vi "运维调试.vi"() -> ()   [LabVIEW 2016]
uses:
  <vilib>/Utility/miscctls.llb/LVPointTypeDef.ctl
  PLC/PLC.lvlib
  API/CodCr/CodCr.lvlib
  <vilib>/Utility/config.llb/NI_LVConfig.lvlib
panel:
  out "数值":i32
  in  "运维调试菜单":T1(xcontrol)
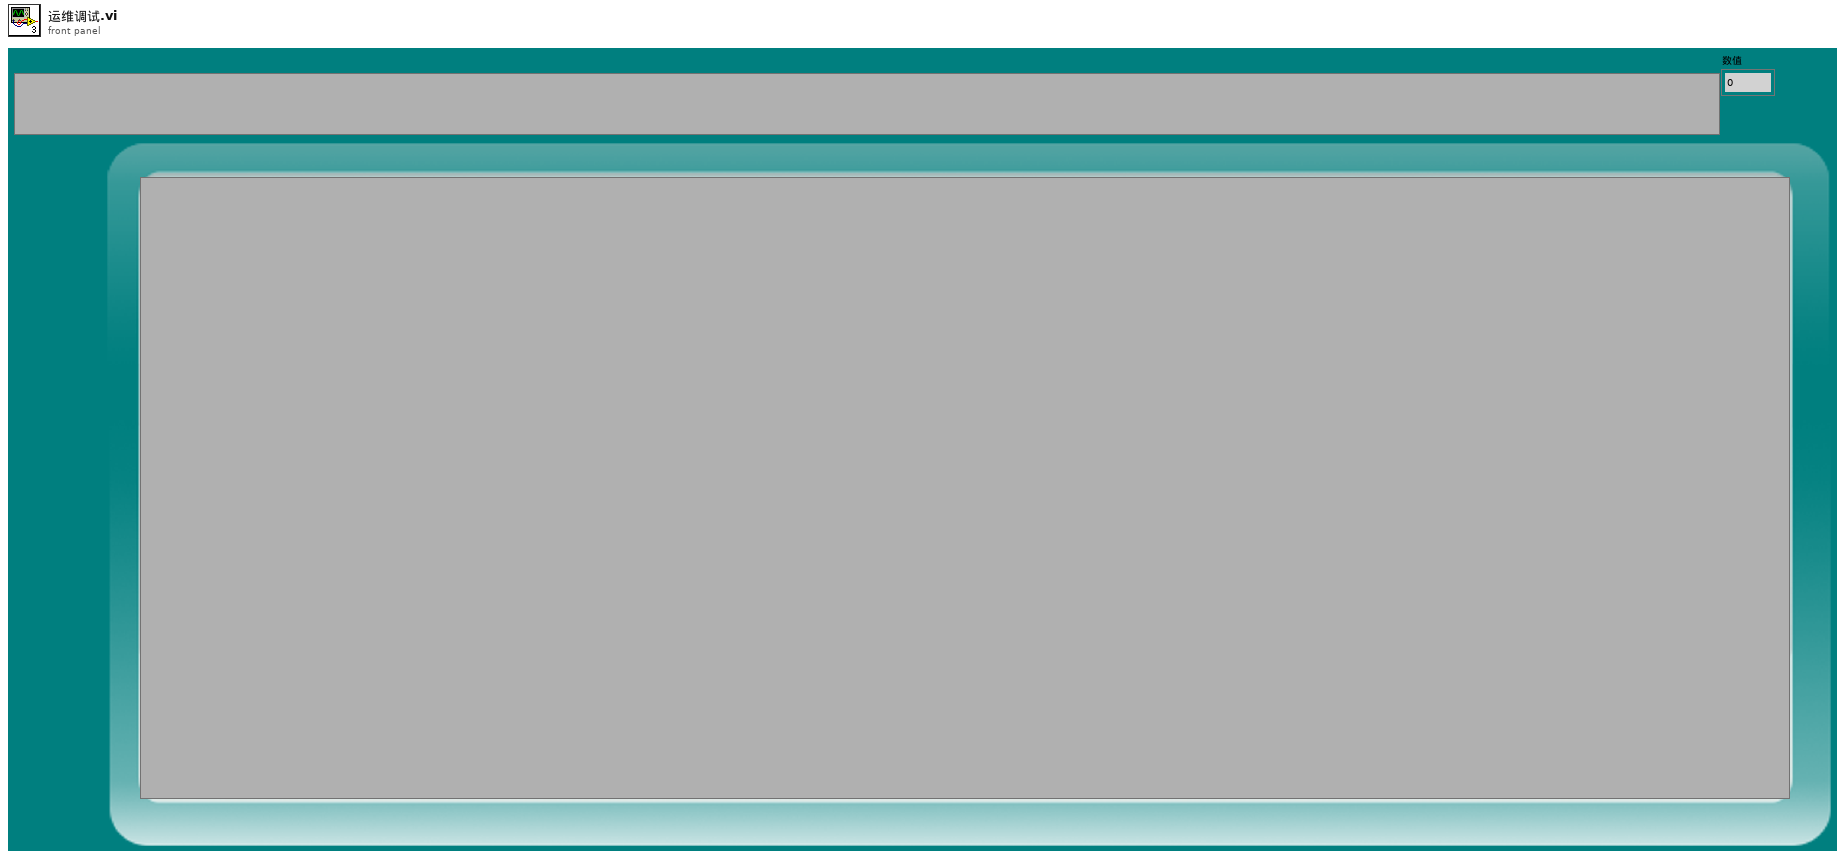
[diagram p1: front panel]
types:
  T1 = enum16{"电源管理", "采配水", "氨氮", "总磷总氮", "多参数", "CODMn", "CODcr", "流量计", "质控单元", "其他"}
  T2 = typedef "NI_LVConfig.lvlib/Config Data RefNum.ctl" = refnum<k1>
  T3 = typedef "LVPointTypeDef.ctl" = cluster{"Horizontal":i16, "Vertical":i16}
  T4 = enum16{"Enabled", "Disabled", "Disabled and Grayed Out"}
  T5 = enum32{"Bad", "Idle", "Run top level", "Running"}
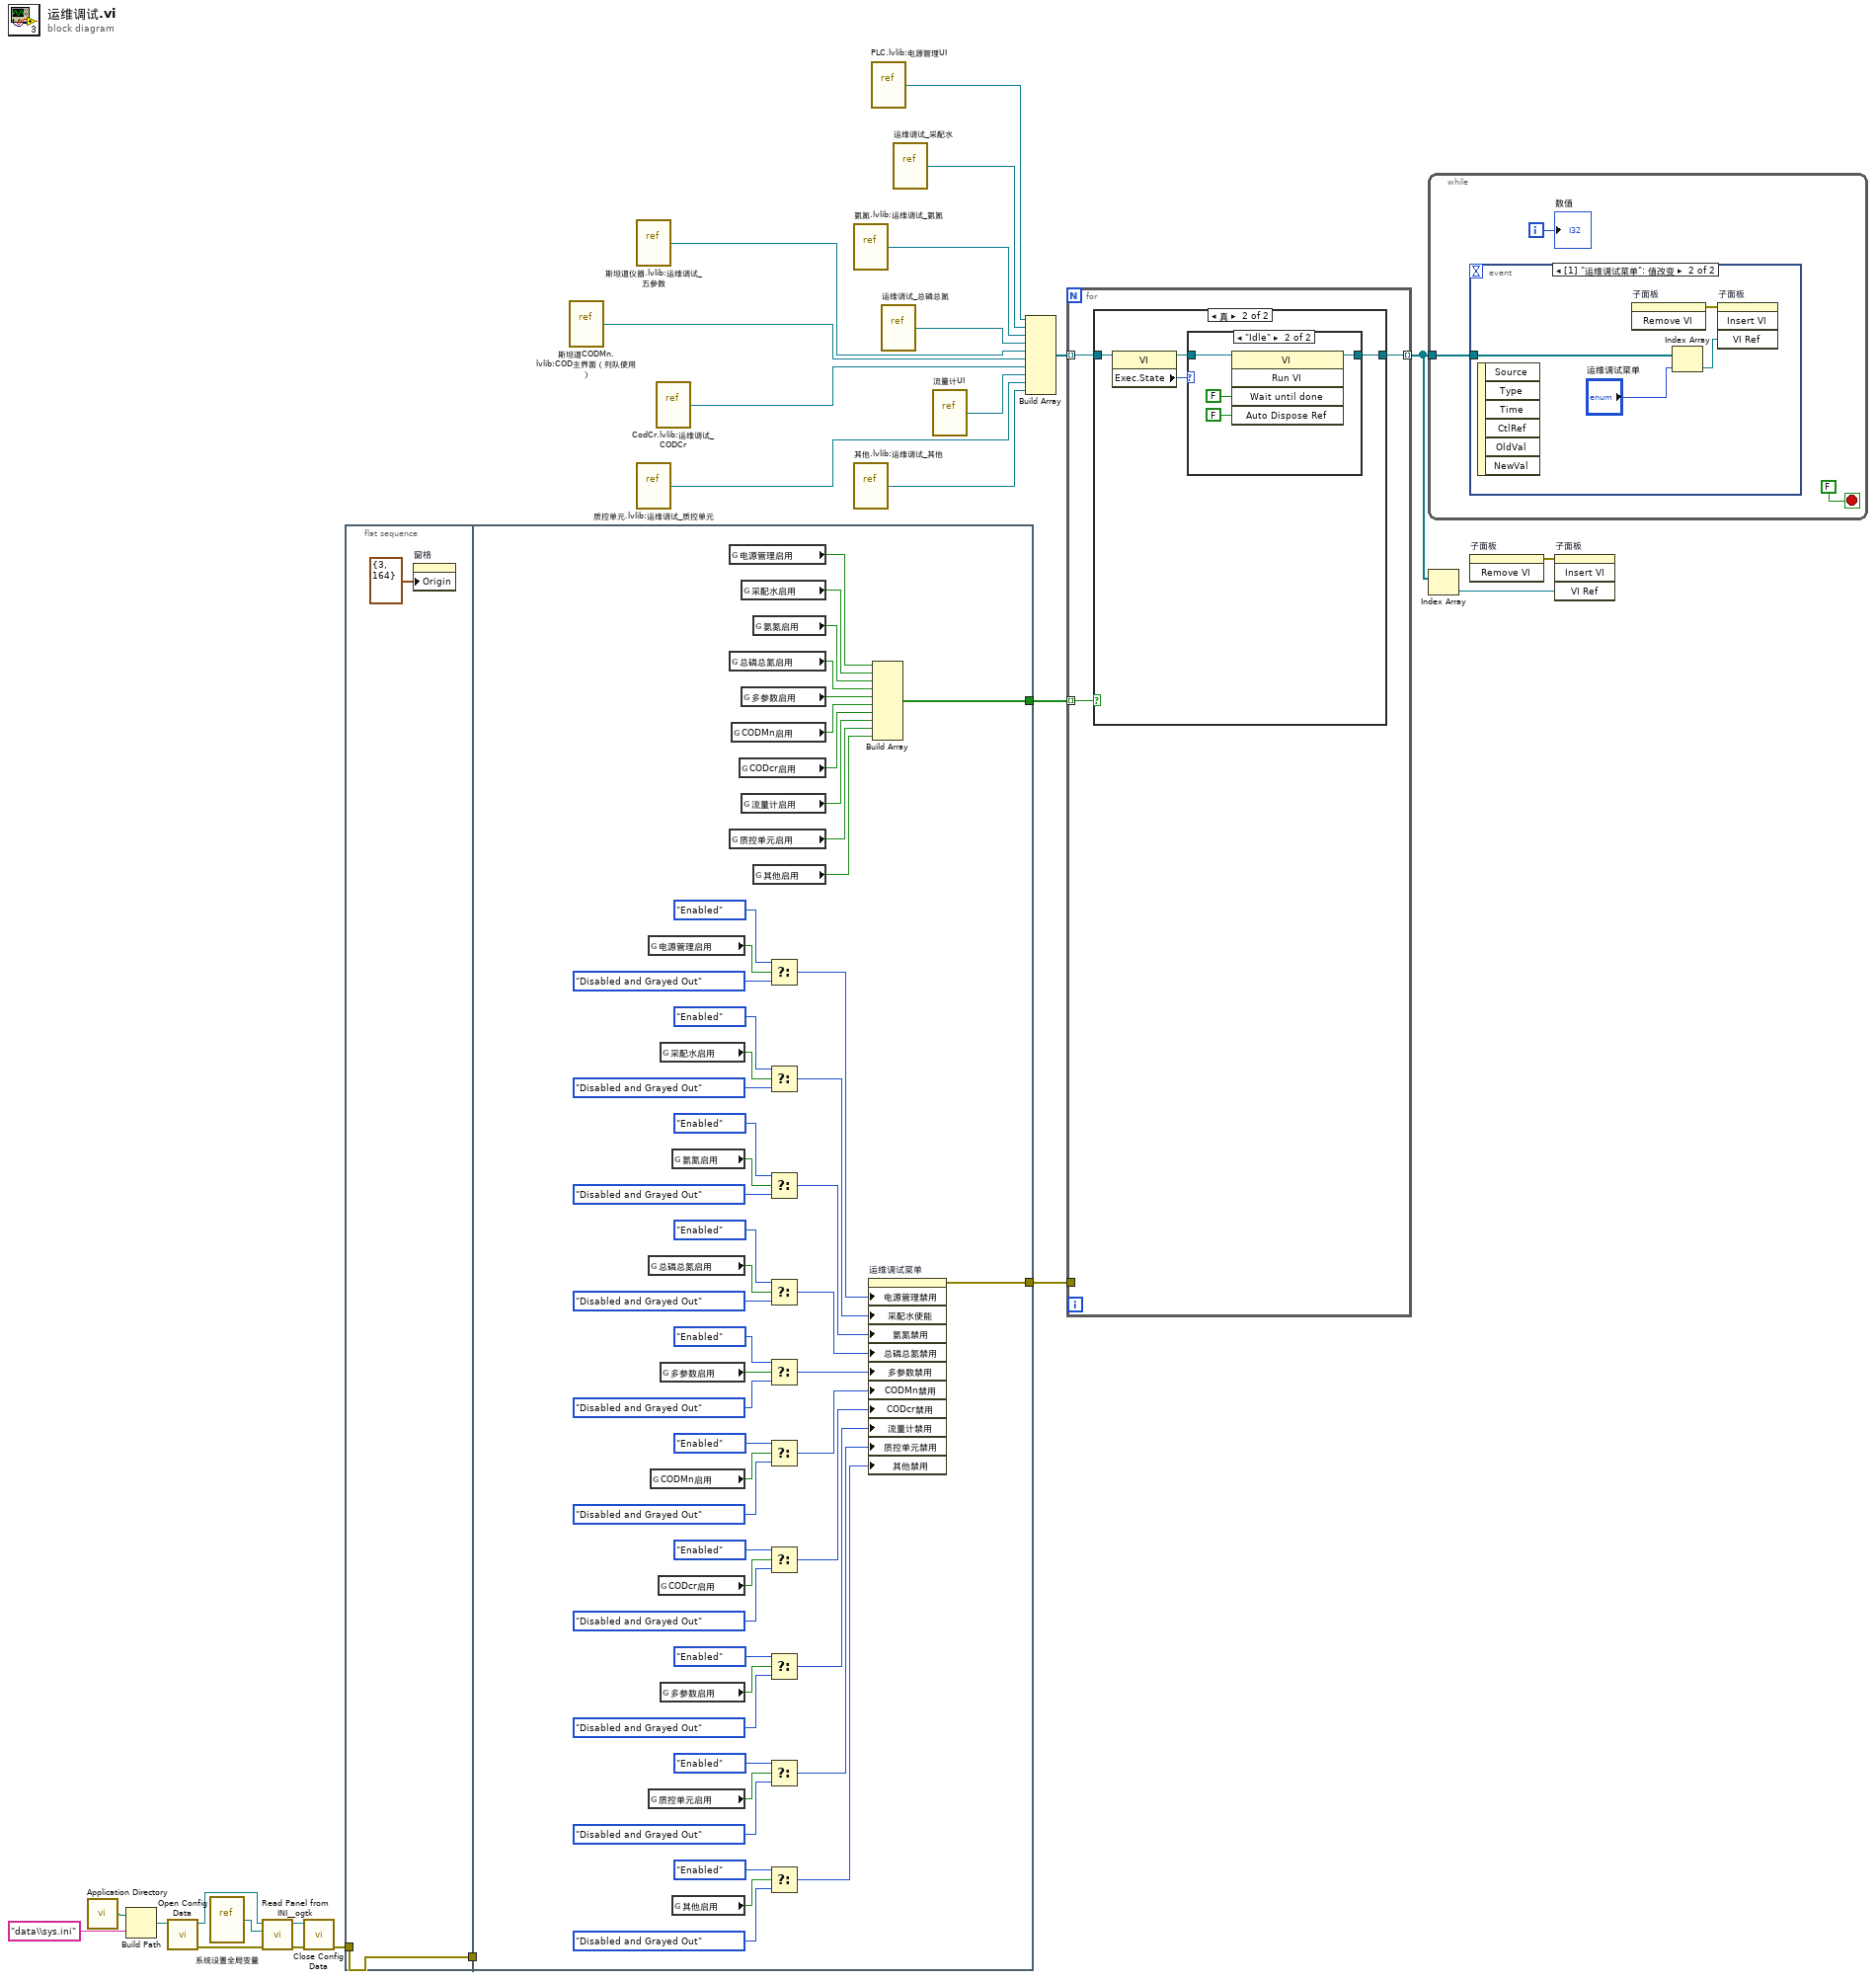
[diagram p0: block diagram]
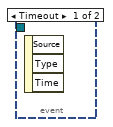
[diagram p4: hidden frame]
diagram:
  n1 = call <vilib>:"Application Directory.vi"() -> ("Application Directory"=w4:path)
  n2 = Build Path(base path=w4, name or relative path="data\\sys.ini" ("名称或相对路径")) -> (appended path=w2:path)
  n3 = call <vilib>:"Open Config Data.vi"("configuration file path"=w2) -> ("error out"=w11:errorcluster, "refnum"=w10:T2)  [unwired: 8 in, 1 out]
  n4 = vi-ref "系统设置全局变量.vi"() -> (w9:refnum<vi>)
  n5 = call <userlib>:"Read Panel from INI__ogtk.vi"("error in (no error)"=w11, "VI ref"=w9, "refnum"=w10) -> ("error out"=w8:errorcluster, "refnum out"=w7:T2)  [unwired: 7 in]
  n6 = call <vilib>:"Close Config Data.vi"("error in (no error)"=w8, "refnum"=w7) -> ("error out"=w6:errorcluster)  [unwired: 8 in, 1 out]
  n7 = flat-sequence {
    tunnel: w6 -> [w28]
    tunnel: [w28] -> w5
    tunnel: [w60] -> w12
    tunnel: w5 -> [_]
    tunnel: [w49] -> w1
    frame #0 {
      n8 = property on="窗格" class="Pane"("Origin"=T3 {"Horizontal"=3, "Vertical"=164} ("原点")) -> ()  [unwired: 2 in, 2 out]
    }
    frame #1 {
      n9 = global read "系统设置全局变量.vi" "电源管理启用"() -> (w80:bool)
      n10 = global read "系统设置全局变量.vi" "总磷总氮启用"() -> (w74:bool)
      n11 = global read "系统设置全局变量.vi" "质控单元启用"() -> (w67:bool)
      n12 = global read "系统设置全局变量.vi" "CODMn启用"() -> (w70:bool)
      n13 = global read "系统设置全局变量.vi" "CODcr启用"() -> (w69:bool)
      n14 = global read "系统设置全局变量.vi" "采配水启用"() -> (w77:bool)
      n15 = global read "系统设置全局变量.vi" "多参数启用"() -> (w72:bool)
      n16 = global read "系统设置全局变量.vi" "多参数启用"() -> (w68:bool)
      n17 = global read "系统设置全局变量.vi" "氨氮启用"() -> (w76:bool)
      n18 = global read "系统设置全局变量.vi" "其他启用"() -> (w66:bool)
      n19 = global read "系统设置全局变量.vi" "电源管理启用"() -> (w50:bool)
      n20 = global read "系统设置全局变量.vi" "总磷总氮启用"() -> (w53:bool)
      n21 = global read "系统设置全局变量.vi" "质控单元启用"() -> (w58:bool)
      n22 = global read "系统设置全局变量.vi" "CODMn启用"() -> (w55:bool)
      n23 = global read "系统设置全局变量.vi" "CODcr启用"() -> (w56:bool)
      n24 = global read "系统设置全局变量.vi" "采配水启用"() -> (w51:bool)
      n25 = global read "系统设置全局变量.vi" "多参数启用"() -> (w54:bool)
      n26 = global read "系统设置全局变量.vi" "流量计启用"() -> (w57:bool)
      n27 = global read "系统设置全局变量.vi" "氨氮启用"() -> (w52:bool)
      n28 = global read "系统设置全局变量.vi" "其他启用"() -> (w59:bool)
      n29 = Select(t=T4."Enabled" ("电源管理禁用"), s=w80, f=T4."Disabled and Grayed Out" ("电源管理禁用")) -> (s? t:f=w79:T4)
      n30 = Select(t=T4."Enabled" ("电源管理禁用"), s=w77, f=T4."Disabled and Grayed Out" ("电源管理禁用")) -> (s? t:f=w78:T4)
      n31 = Select(t=T4."Enabled" ("电源管理禁用"), s=w76, f=T4."Disabled and Grayed Out" ("电源管理禁用")) -> (s? t:f=w75:T4)
      n32 = Select(t=T4."Enabled" ("电源管理禁用"), s=w74, f=T4."Disabled and Grayed Out" ("电源管理禁用")) -> (s? t:f=w73:T4)
      n33 = Select(t=T4."Enabled" ("电源管理禁用"), s=w72, f=T4."Disabled and Grayed Out" ("电源管理禁用")) -> (s? t:f=w71:T4)
      n34 = Select(t=T4."Enabled" ("电源管理禁用"), s=w70, f=T4."Disabled and Grayed Out" ("电源管理禁用")) -> (s? t:f=w65:T4)
      n35 = Select(t=T4."Enabled" ("电源管理禁用"), s=w69, f=T4."Disabled and Grayed Out" ("电源管理禁用")) -> (s? t:f=w64:T4)
      n36 = Select(t=T4."Enabled" ("电源管理禁用"), s=w68, f=T4."Disabled and Grayed Out" ("电源管理禁用")) -> (s? t:f=w63:T4)
      n37 = Select(t=T4."Enabled" ("电源管理禁用"), s=w67, f=T4."Disabled and Grayed Out" ("电源管理禁用")) -> (s? t:f=w62:T4)
      n38 = Select(t=T4."Enabled" ("电源管理禁用"), s=w66, f=T4."Disabled and Grayed Out" ("电源管理禁用")) -> (s? t:f=w61:T4)
      n39 = property on="运维调试菜单" class="运维调试菜单 (严格)"("电源管理禁用"=w79, "采配水使能"=w78, "氨氮禁用"=w75, "总磷总氮禁用"=w73, "多参数禁用"=w71, "CODMn禁用"=w65, "CODcr禁用"=w64, "流量计禁用"=w63, "质控单元禁用"=w62, "其他禁用"=w61) -> (error out=w60:errorcluster)  [unwired: 2 in, 1 out]
      n40 = Build Array(w50, w51, w52, w53, w54, w55, w56, w57, w58, w59) -> (w49:bool[])
    }
  }
  n41 = vi-ref "斯坦道CODMn.lvlib:COD主界面（列队使用）.vi"() -> (w18:refnum<vi>)
  n42 = vi-ref "斯坦道仪器.lvlib:运维调试_五参数.vi"() -> (w19:refnum<vi>)
  n43 = vi-ref "质控单元.lvlib:运维调试_质控单元.vi"() -> (w16:refnum<vi>)
  n44 = vi-ref "CodCr.lvlib:运维调试_CODCr.vi"() -> (w17:refnum<vi>)
  n45 = vi-ref "氨氮.lvlib:运维调试_氨氮.vi"() -> (w21:refnum<vi>)
  n46 = vi-ref "其他.lvlib:运维调试_其他.vi"() -> (w15:refnum<vi>)
  n47 = vi-ref "PLC.lvlib:电源管理UI.vi"() -> (w14:refnum<vi>)
  n48 = vi-ref "运维调试_总磷总氮.vi"() -> (w20:refnum<vi>)
  n49 = vi-ref "运维调试_采配水.vi"() -> (w22:refnum<vi>)
  n50 = vi-ref "流量计UI.vi"() -> (w13:refnum<vi>)
  n51 = Build Array(w14, w22, w21, w20, w19, w18, w17, w13, w16, w15) -> (w23:refnum<vi>[])
  n52 = for {
    tunnel: w23 -> [w83] mode=indexing
    tunnel: [w82] -> w25 mode=indexing
    tunnel: w1 -> [w81] mode=indexing
    tunnel: w12 -> [_]
    n53 = case shown="真" w81 {
      tunnel: w83 -> [w84 w88]
      tunnel: [w84 w85] -> w82
      frame False {
      }
      frame True {
        n54 = property class="VI"(reference=w88) -> (reference out=w86:refnum<vi>, "Exec.State"=w87:T5)  [unwired: 1 in, 1 out]
        n55 = case shown="\"Idle\"" w87 {
          tunnel: w86 -> [w89 w91]
          tunnel: [w89 w90] -> w85
          frame "Bad", Default {
          }
          frame "Idle" {
            n56 = invoke class="VI" method="Run VI"(reference=w91, "Wait until done"=FALSE ("结束前等待"), "Auto Dispose Ref"=FALSE ("自动销毁引用")) -> (reference out=w90:refnum<vi>)  [unwired: 2 in, 4 out]
          }
        }
      }
    }
  }
  n57 = while {
    tunnel: w25 -> [w95]
    i -> [w94]
    stop <- FALSE stop-if-true
    n58 = event shown="[1] \"运维调试菜单\": 值改变" {
      selector: _ -> [_ _]
      dyn-events: _ -> [_ _]
      timeout: _ -> [_ _]
      tunnel: w95 -> [_ w99]
      event Timeout {
        n59 = event-data() -> ()  [unwired: 1 in, 3 out]
      }
      event "运维调试菜单": Value Change {
        n60 = event-data() -> ()  [unwired: 1 in, 6 out]
        n61 = invoke on="子面板" class="SubPnl" method="Remove VI"() -> (error out=w100:errorcluster)  [unwired: 3 in, 2 out]
        n62 = Index Array(array=w99, index="运维调试菜单") -> (element=w98:refnum<vi>)
        n63 = invoke on="子面板" class="SubPnl" method="Insert VI"(error in=w100, "VI Ref"=w98) -> ()  [unwired: 2 in, 4 out]
      }
    }
    "数值" <- w94
  }
  n64 = Index Array(array=w25) -> (element=w24:refnum<vi>)  [unwired: 1 in]
  n65 = invoke on="子面板" class="SubPnl" method="Remove VI"() -> (error out=w26:errorcluster)  [unwired: 3 in, 2 out]
  n66 = invoke on="子面板" class="SubPnl" method="Insert VI"(error in=w26, "VI Ref"=w24) -> ()  [unwired: 2 in, 4 out]
